vi "Parameters FG.vi"(6 "Params Operations (Get)":T4=enum."Get", 7 "configuration file path":path=path "d:/Test.vi", 8 "error in":errorcluster, 11 "MultiScale Parameters In":T1={"Preprocessing"=enum."Do Not Process", "Convolution"=enum."Seifert 5x5", "Unsharp Mask Params"={"Amount"=6.0, "Radius"=33.0, "Threshold"=30.0}, "LUT Power"=[0.61538464, 0.43076923, 0.3846154, 0.43846154, 0.42307693, 0.5538462, 0.64615387, 0.61538464, 0.61538464, 0.6, 0.4, 0.4], "LUT Multiplier"=[157.53847, 185.1077, 192.98462, 248.12308, 196.92308, 248.12308, 252.06154, 114.215385, 248.12308, 110.276924, 102.4, 102.4], "Filters"=[enum."Seifert 7x7", enum."Seifert 5x5", enum."Highlight Details 3x3", enum."None", enum."None", enum."None", enum."None", enum."None", enum."None", enum."None", enum."None", enum."None"], "X Value PostProc"=1.2} {"X Value PostProc" scale=0.75..3.0; "LUT Multiplier" scale=0.0..512.0; "LUT Power" scale=0.0..2.0}) -> (0 "error out":errorcluster, 3 "MultiScale Parameters Out":T1={"Preprocessing"=enum."Do Not Process", "Convolution"=enum."Seifert 5x5", "Unsharp Mask Params"={"Amount"=6.0, "Radius"=33.0, "Threshold"=30.0}, "LUT Power"=[0.61538464, 0.43076923, 0.3846154, 0.43846154, 0.42307693, 0.5538462, 0.64615387, 0.61538464, 0.61538464, 0.6, 0.4, 0.4], "LUT Multiplier"=[157.53847, 185.1077, 192.98462, 248.12308, 196.92308, 248.12308, 252.06154, 114.215385, 248.12308, 110.276924, 102.4, 102.4], "Filters"=[enum."Seifert 7x7", enum."Seifert 5x5", enum."Highlight Details 3x3", enum."None", enum."None", enum."None", enum."None", enum."None", enum."None", enum."None", enum."None", enum."None"], "X Value PostProc"=1.2} {"X Value PostProc" scale=0.75..3.0; "LUT Multiplier" scale=0.0..512.0; "LUT Power" scale=0.0..2.0})   [LabVIEW 2023]
uses:
  Multiscale Parameters Typedef.ctl
  Conv Flt Presets.ctl
  Unsharp Mask Params TypeDef.ctl
  Parameters Operations.ctl
  <vilib>/Utility/config.llb/NI_LVConfig.lvlib
panel:
  # "1024x1024"
  # "2048x2048"
  # "4096x4096"
  # "1024x1024"
  # "2048x2048"
  # "4096x4096"
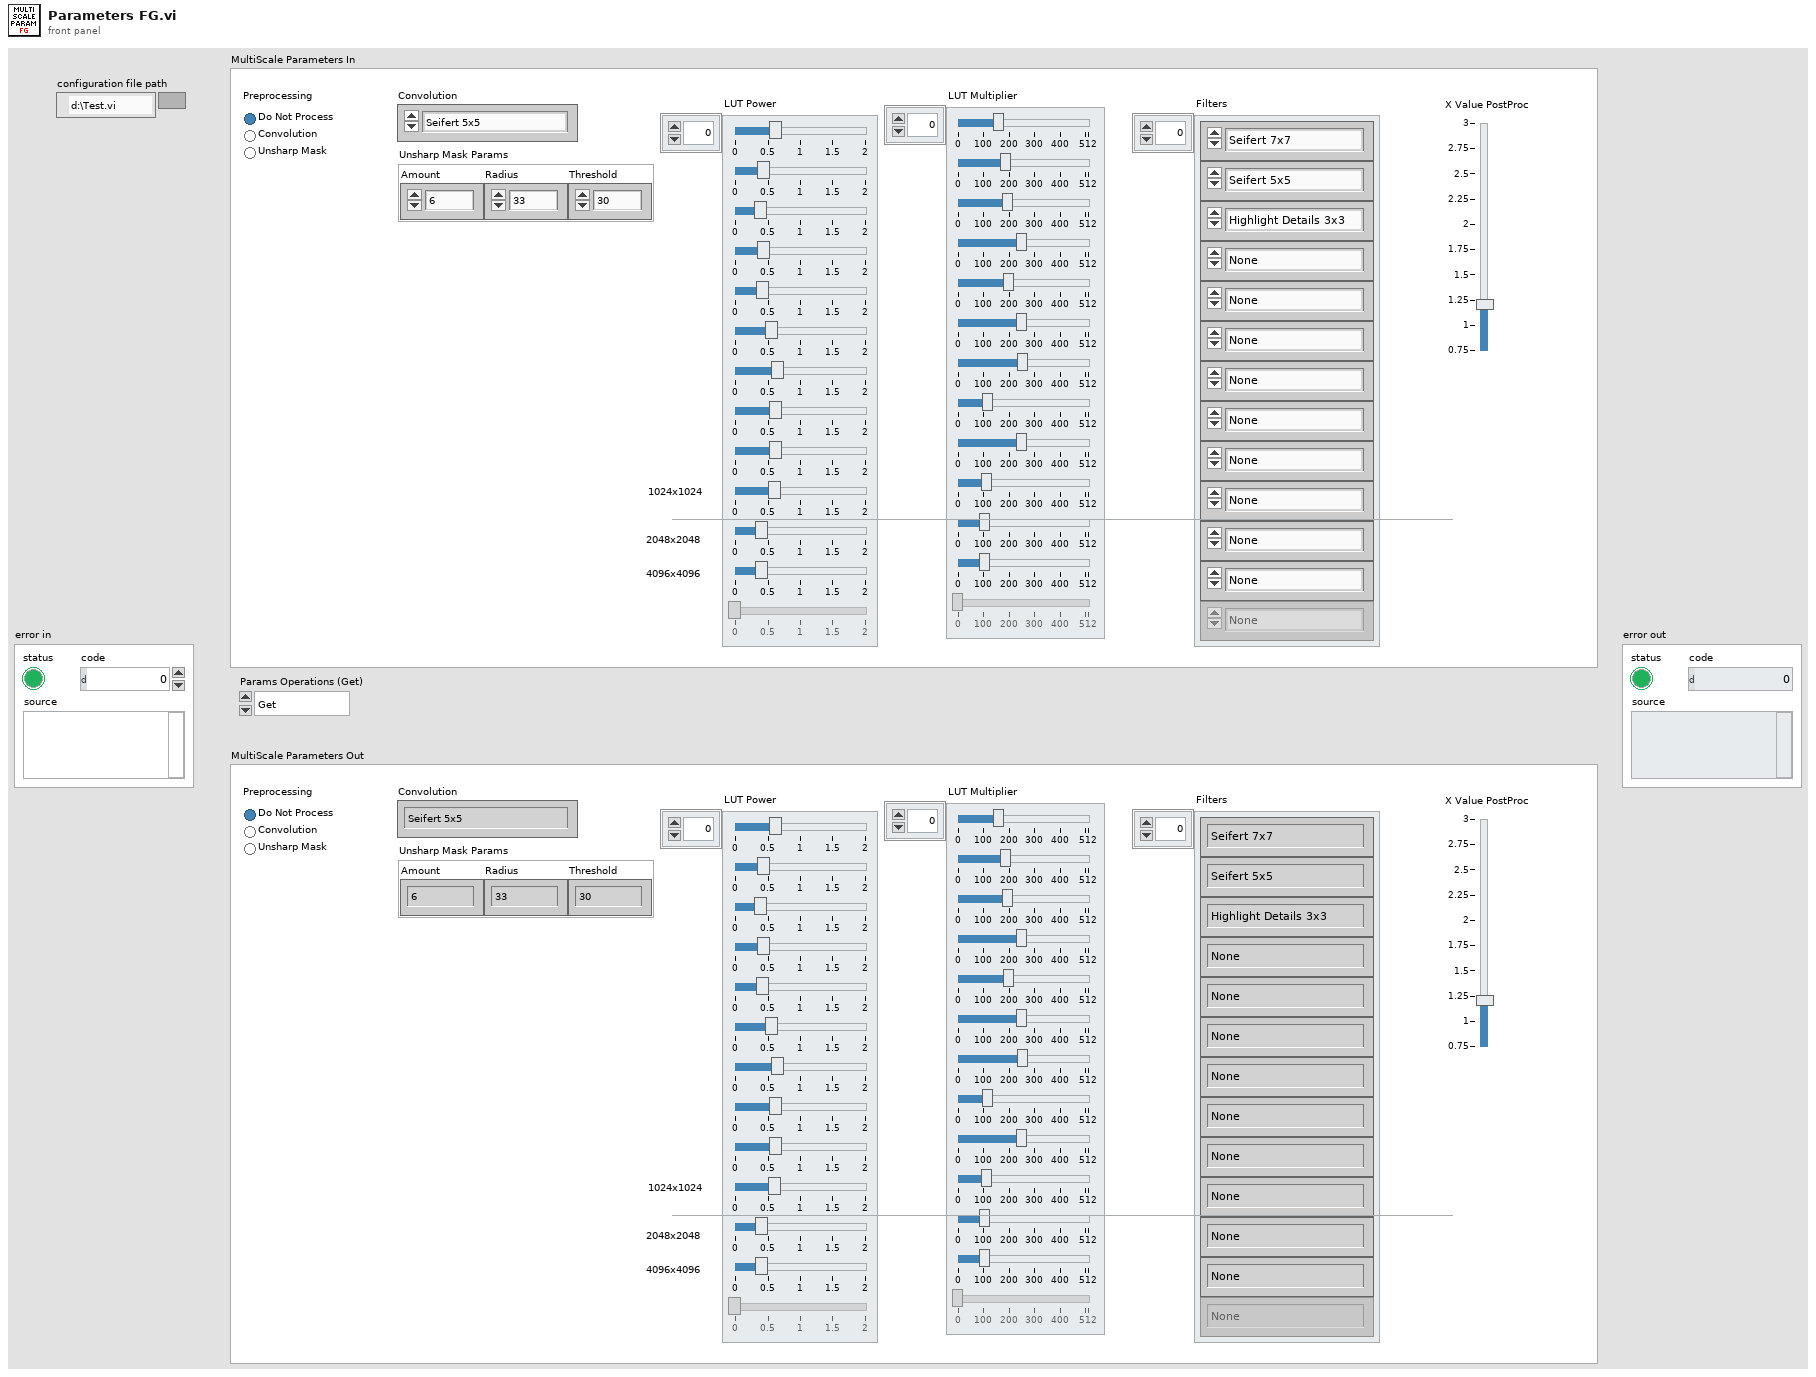
[diagram p1: front panel]
types:
  T1 = typedef "Multiscale Parameters Typedef.ctl" = cluster{"Preprocessing":enum32{"Do Not Process", "Convolution", "Unsharp Mask"}, "Convolution":T2, "Unsharp Mask Params":T3, "LUT Power":sgl[], "LUT Multiplier":sgl[], "Filters":T2[], "X Value PostProc":sgl}
  T2 = typedef "Conv Flt Presets.ctl" = enum16{"None", "Seifert 5x5", "Seifert 7x7", "High Pass 5x5 ", "High Pass 7x7", "Highlight Details 3x3", "Highlight Details 5x5", "Highlight Detail 7x7"}
  T3 = typedef "Unsharp Mask Params TypeDef.ctl" = cluster{"Amount":sgl, "Radius":sgl, "Threshold":sgl}
  T4 = typedef "Parameters Operations.ctl" = enum16{"Init", "Get", "Apply", "Save to File", "Load from File"}
  T5 = typedef "NI_LVConfig.lvlib/Config Data RefNum.ctl" = refnum<k1>
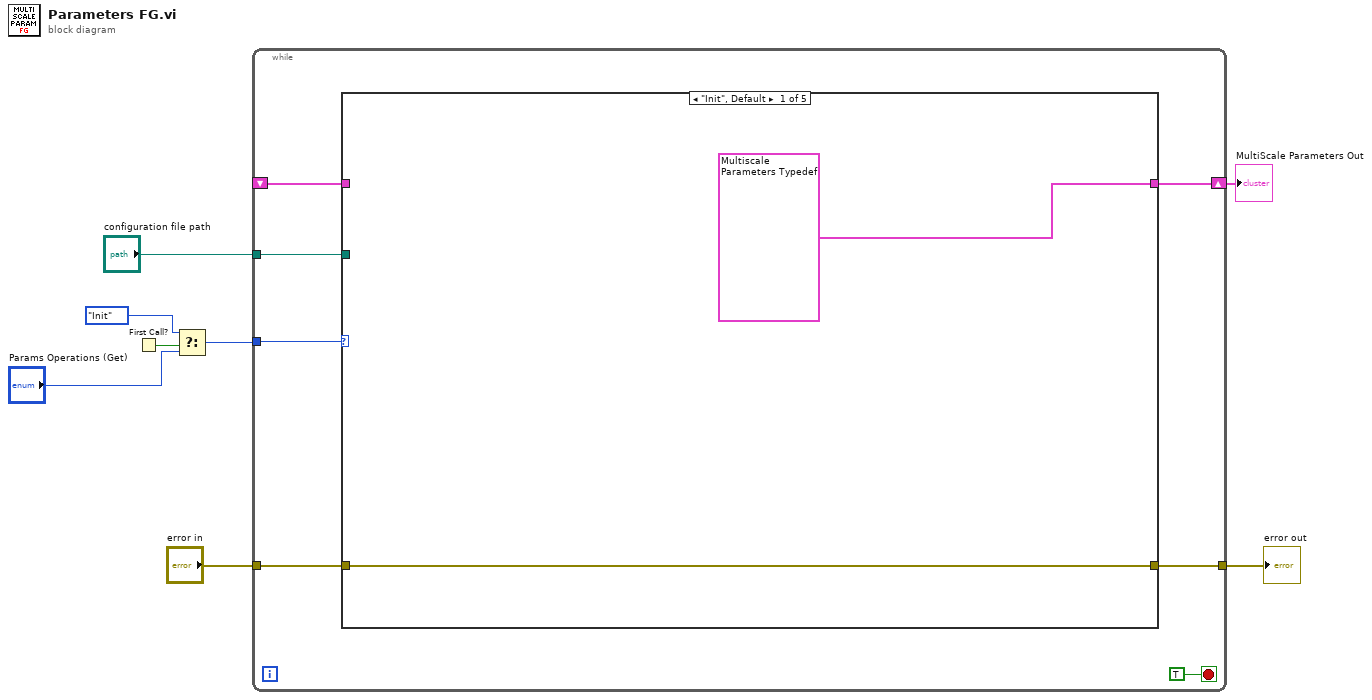
[diagram p0: block diagram]
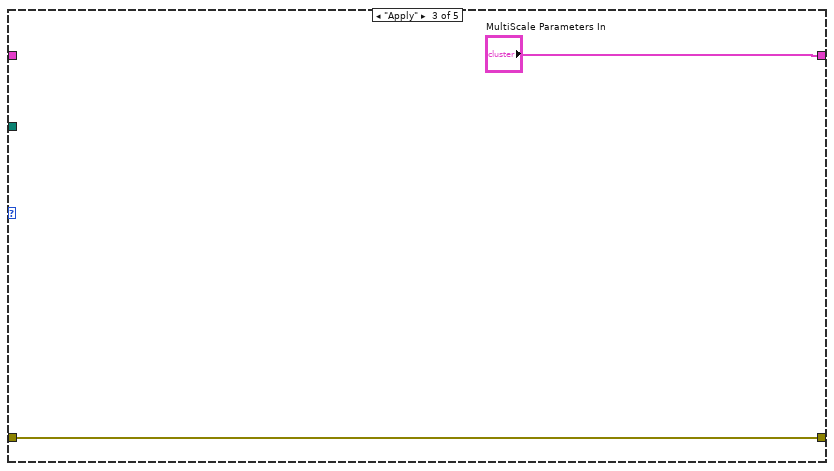
[diagram p3: hidden frame]
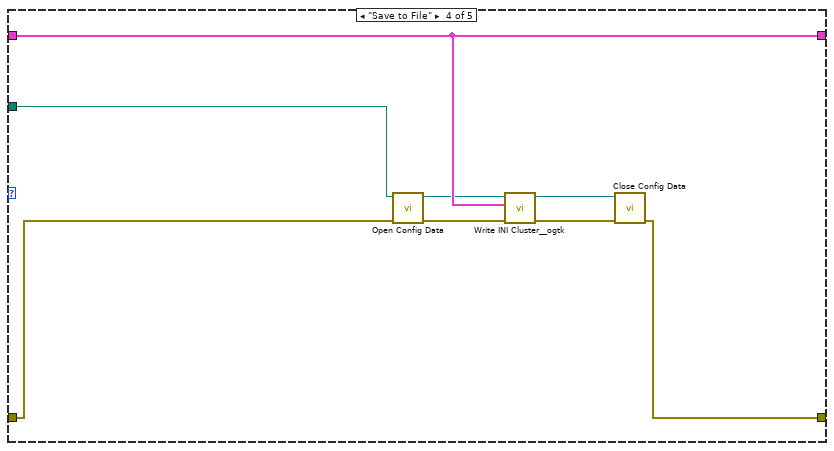
[diagram p4: hidden frame]
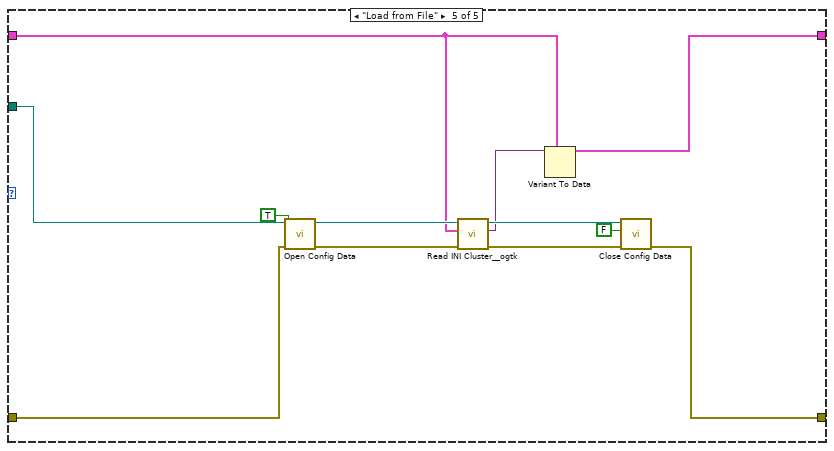
[diagram p5: hidden frame]
diagram:
  n1 = First Call?() -> (First Call?: T/F=w5:bool)
  n2 = Select(t=Parameters_Operations."Init" ("Params Operations"), s=w5, f="Params Operations (Get)") -> (s? t:f=w2:T4)
  n3 = while {
    shift-right: [w14] -> w8
    shift-left: _ -> [w13]
    tunnel: w2 -> [w12]
    tunnel: "error in" -> [w11]
    tunnel: [w10] -> w6
    tunnel: "configuration file path" -> [w9]
    stop <- TRUE stop-if-true
    n4 = case shown="\"Init\", Default" w12 {
      tunnel: [T1 {"Preprocessing"=enum."Convolution", "Convolution"=enum."Seifert 5x5", "Unsharp Mask Params"={"Amount"=6.0, "Radius"=33.0, "Threshold"=30.0}, "LUT Power"=[0.5846154, 0.43076923, 0.3846154, 0.43846154, 0.42307693, 0.5538462, 0.64615387, 0.61538464, 0.61538464, 0.6, 0.4, 0.4], "LUT Multiplier"=[177.23077, 212.67693, 153.6, 248.12308, 196.92308, 248.12308, 252.06154, 114.215385, 248.12308, 110.276924, 102.4, 102.4], "Filters"=[enum."None", enum."Seifert 5x5", enum."Highlight Details 3x3", enum."None", enum."None", enum."None", enum."None", enum."None", enum."None", enum."None", enum."None", enum."None"], "X Value PostProc"=1.2059472} ("MultiScale Parameters") w19 "MultiScale Parameters In" w29 w35] -> w14
      tunnel: w13 -> [_ w19 _ w29 w36]
      tunnel: w11 -> [w16 w18 w20 w26 w34]
      tunnel: [w16 w18 w20 w23 w31] -> w10
      tunnel: w9 -> [_ _ _ w22 w30]
      frame "Init", Default {
      }
      frame "Get" {
      }
      frame "Apply" {
      }
      frame "Save to File" {
        n5 = call <vilib>:"Open Config Data.vi"("error in (no error)"=w26, "configuration file path"=w22) -> ("error out"=w25:errorcluster, "refnum"=w28:T5)  [unwired: 7 in, 1 out]
        n6 = call <userlib>:"Write INI Cluster__ogtk.vi"("error in (no error)"=w25, "INI Fomatted Cluster"=w29, "refnum"=w28) -> ("error out"=w24:errorcluster, "dup refnum"=w27:T5)  [unwired: 7 in]
        n7 = call <vilib>:"Close Config Data.vi"("error in (no error)"=w24, "refnum"=w27) -> ("error out"=w23:errorcluster)  [unwired: 8 in, 1 out]
      }
      frame "Load from File" {
        n8 = call <vilib>:"Open Config Data.vi"("error in (no error)"=w34, "create file if necessary (T)"=TRUE, "configuration file path"=w30) -> ("error out"=w33:errorcluster, "refnum"=w39:T5)  [unwired: 6 in, 1 out]
        n9 = call <userlib>:"Read INI Cluster__ogtk.vi"("error in (no error)"=w33, "INI Fomatted Cluster Type"=w36, "refnum"=w39) -> ("error out"=w32:errorcluster, "INI Fomatted Cluster"=w37:variant, "dup refnum"=w41:T5)  [unwired: 4 in, 2 out]
        n10 = Variant To Data(type=w36, Variant=w37) -> (data=w35:T1)  [unwired: 1 in, 1 out]
        n11 = call <vilib>:"Close Config Data.vi"("error in (no error)"=w32, "write file if changed (T)"=FALSE, "refnum"=w41) -> ("error out"=w31:errorcluster)  [unwired: 7 in, 1 out]
      }
    }
  }
  "MultiScale Parameters Out" <- w8
  "error out" <- w6
